vi "Conditionally Add SDI Parameter.vi"(10 "create SDI (F)":bool, 11 "parameters in":T1[](array[typedef])) -> (3 "parameters out":T1[](array[typedef]))   [LabVIEW 2020]
uses:
  VS Channel Definition for Parameter.ctl
  Direction.ctl
  Parameter Definition.ctl
  Encoding and Decoding/Encoding.ctl
  Encoding and Decoding/Encoding and Decoding.lvlib
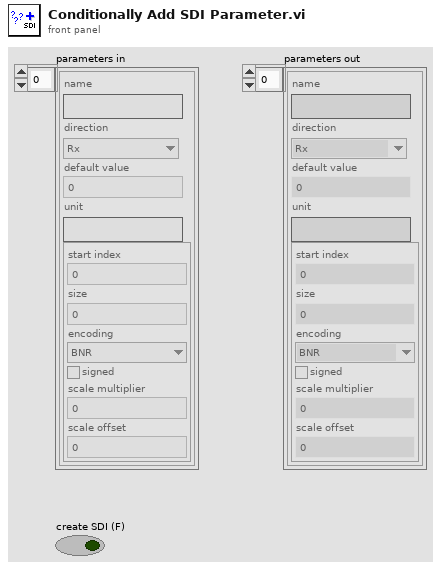
[diagram p1: front panel]
types:
  T1 = typedef "VS Channel Definition for Parameter.ctl" = cluster{"name":string, "direction":T2, "default value":dbl, "unit":string, "Parameter":T3}
  T2 = typedef "Direction.ctl" = enum16{"Rx", "Tx"}
  T3 = typedef "Parameter Definition.ctl" = cluster{"start index":i32, "size":i32, "encoding":T4, "signed":bool, "scale multiplier":dbl, "scale offset":dbl}
  T4 = typedef "Encoding and Decoding.lvlib/Encoding.ctl" = enum16{"BNR", "BCD", "Discrete"}
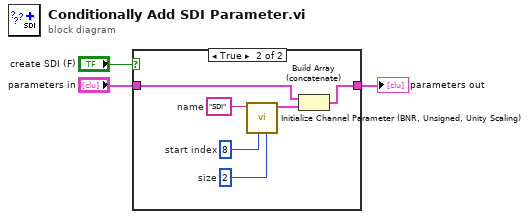
[diagram p0: block diagram]
diagram:
  n1 = case shown="True" "create SDI (F)" {
    tunnel: "parameters in" -> [w4 w10]
    tunnel: [w4 w9] -> w3
    frame False {
    }
    frame True {
      w8 = 2  # size
      w7 = 8  # start index
      w6 = "SDI"  # name
      n2 = call "Initialize Channel Parameter (BNR, Unsigned, Unity Scaling).vi"("size"=w8, "start index"=w7, "name"=w6) -> ("channel parameter"=w5:T1)  [unwired: 8 in]
      n3 = Build Array (concatenate)(w10, w5) -> (w9:T1[])
    }
  }
  "parameters out" <- w3
